vi "Open_QA.vi"(8 "error in (no error)":errorcluster, 11 "URL":string="https://epcpower.odoo.com/web#id=&action=398&active_id=1&model=quality.alert&view_type=form&menu_id=274") -> (0 "error out":errorcluster)   [LabVIEW 2022 SP3]
uses:
  <vilib>/Platform/browser.llb/Open URL in Default Browser (string).vi
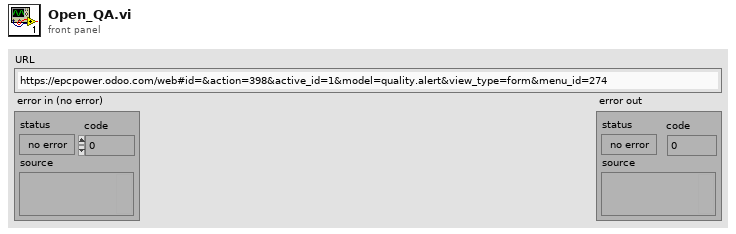
[diagram p1: front panel]
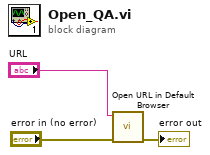
[diagram p0: block diagram]
diagram:
  n1 = call-poly <vilib>:"Open URL in Default Browser.vi"("error in (no error)"="error in (no error)", "URL"="URL") -> ("error out"=→"error out":errorcluster)  [unwired: 4 in, 1 out]
